vi "Dialog.vi"(0 "error handler in":refnum<class "TLB` Error Handler.lvclass">, 5 "trigger queue in":refnum<queue>) -> (4 "error handler out":refnum<class "TLB` Error Handler.lvclass">, 15 "error out":errorcluster)   [LabVIEW 2018, in "Springboard TLB`.lvlib" / "TLB` Error Handler.lvclass"]
doc: "error dialog that users interact with to make decisions based upon capture errors.\n\n<B>Input Parameters</B>\n\n<B>error handler in</B> identifies your session. <B>Error Handler in</B> is obtained from the Open.vi of this class.\n\n<B>MAIN-Trigger Queue in</B> trigger queue reference.\n\n<B>Output Parameters</B>\n\n<B>error handler out</B> identifies your session. <B>Error Handler out</B> is obtained from the Open.vi of this class.\n\n<B>error out</B> contains error information. This output provides standard error out functionality."
uses:
  TLB` Error Handler.lvclass
  Application Components/Trigger API/System Trigger Element.ctl
  Application Components/Trigger API/System Trigger.ctl
  TLB` Error Handler.lvclass/TLB` Error Handler.ctl
  Application Components/Trigger API/Springboard Trigger API.lvlib
panel:
  out "Ring":u16(ring)
  out "source text":string
  in  "Return to Safe State":bool
  in  "error in":errorcluster
  in  "Stop Acquisition":bool
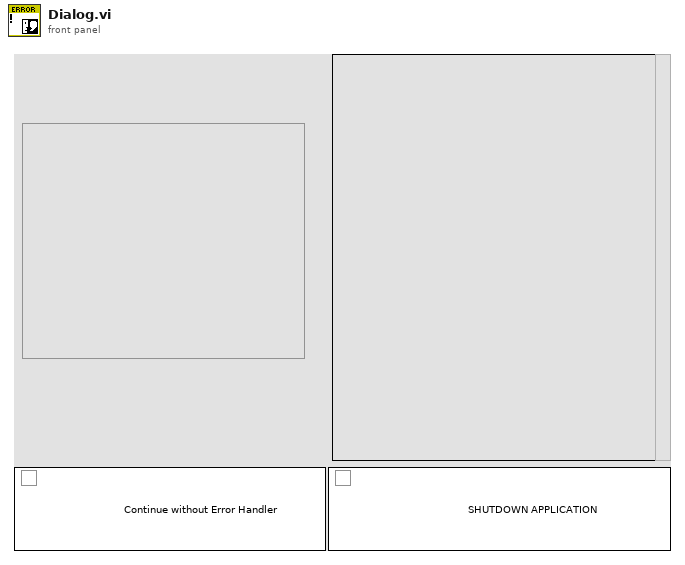
[diagram p1: front panel]
types:
  T1 = typedef "Springboard TLB`.lvlib/Springboard Trigger API.lvlib/System Trigger.ctl" = enum16{"<None>", "<Return to Safe State Actions>", "<Cache User Parameters>", "<Close Application>", "<Error>", "Create New", "Cancel"}
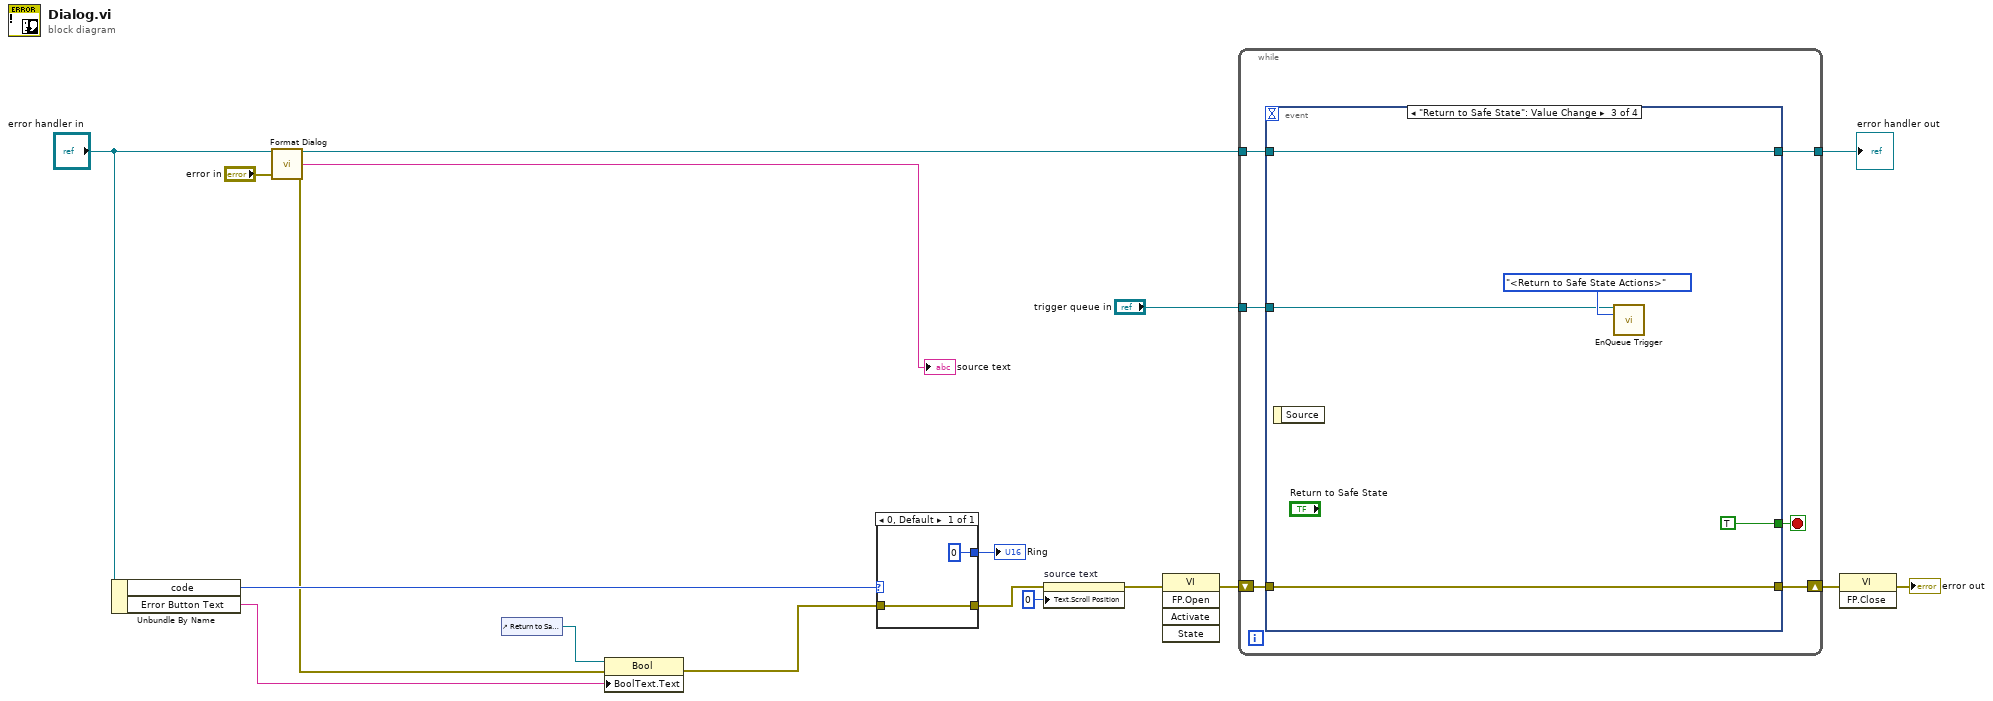
[diagram p0: block diagram]
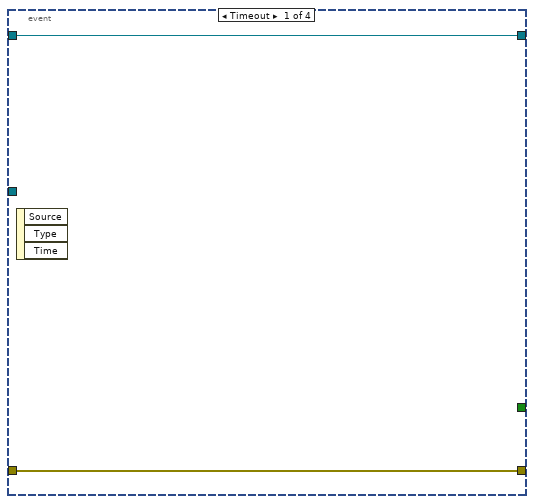
[diagram p2: hidden frame]
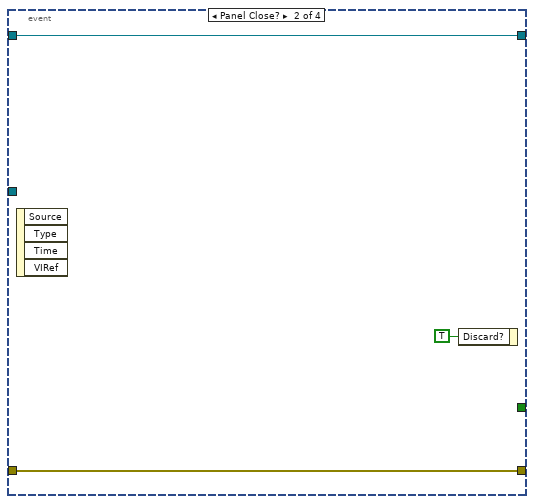
[diagram p3: hidden frame]
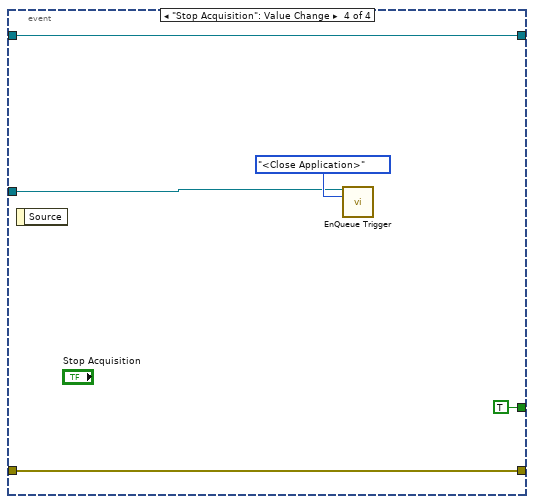
[diagram p4: hidden frame]
diagram:
  n1 = Unbundle By Name("error handler in") -> ("code"=w8:i32, "Error Button Text"=w2:string)
  n2 = call-dynamic "Format Dialog.vi"("error handler in"="error handler in", "error in"="error in") -> ("error handler out"=w6:refnum<class "TLB` Error Handler.lvclass">, "source text"=→"source text":string, "error out"=w3:errorcluster)  [unwired: 11 in]
  n3 = control-ref of="Return to Safe State"() -> (w10:refnum<vi>)
  n4 = property class="Bool"(reference=w10, error in=w3, "BoolText.Text"=w2) -> (error out=w9:errorcluster)  [unwired: 1 out]
  n5 = case shown="0, Default" w8 {
    tunnel: [u16 0 ("Ring")] -> w17
    tunnel: w9 -> [w19]
    tunnel: [w19] -> w13
    frame 0, Default {
    }
  }
  "Ring" <- w17
  n6 = property on="source text" class="Str"(error in=w13, "Text.Scroll Position"=u32 0) -> (error out=w12:errorcluster)  [unwired: 1 in, 1 out]
  n7 = invoke class="VI" method="FP.Open"(error in=w12) -> (error out=w18:errorcluster)  [unwired: 4 in, 4 out]
  n8 = while {
    shift-right: [w25] -> w16
    shift-left: w18 -> [w26]
    tunnel: w6 -> [w23]
    tunnel: [w22] -> w14
    tunnel: "trigger queue in" -> [w21]
    stop <- w24 stop-if-true
    n9 = event shown="[2] \"Return to Safe State\": Value Change" {
      selector: _ -> [_ _ _ _]
      dyn-events: _ -> [_ _ _ _]
      timeout: _ -> [_ _ _ _]
      tunnel: w26 -> [w28 w30 w36 w41]
      tunnel: [w28 w30 w36 w41] -> w25
      tunnel: [_ _ TRUE TRUE] -> w24
      tunnel: w23 -> [w27 w29 w34 w39]
      tunnel: [w27 w29 w34 w39] -> w22
      tunnel: w21 -> [_ _ w32 w37]
      event Timeout {
        n10 = event-data() -> ()  [unwired: 1 in, 3 out]
      }
      event Panel Close? {
        n11 = event-data() -> ()  [unwired: 1 in, 4 out]
        n12 = event-data("Discard?"=TRUE) -> ()  [unwired: 1 in, 1 out]
      }
      event "Return to Safe State": Value Change {
        n13 = event-data() -> ()  [unwired: 1 in, 1 out]
        n14 = call "EnQueue Trigger.vi"("trigger queue in"=w32, "system trigger"=System_Trigger."<Return to Safe State Actions>" ("System Triggers")) -> ()  [unwired: 12 in, 2 out]
      }
      event "Stop Acquisition": Value Change {
        n15 = event-data() -> ()  [unwired: 1 in, 1 out]
        n16 = call "EnQueue Trigger.vi"("trigger queue in"=w37, "system trigger"=System_Trigger."<Close Application>" ("System Triggers")) -> ()  [unwired: 12 in, 2 out]
      }
    }
  }
  "error handler out" <- w14
  n17 = invoke class="VI" method="FP.Close"(error in=w16) -> (error out=→"error out":errorcluster)  [unwired: 2 in, 2 out]
